vi "Convert Flow Data.vi"(8 "error in (no error)":errorcluster, 10 "register values - 3B":u16[](array[numeric]) format="%.0x", 11 "register values - 3A":u16[](array[numeric]) format="%.0x") -> (0 "error out":errorcluster, 3 "Flow Rate (SCFH)":dbl)   [LabVIEW 2020]
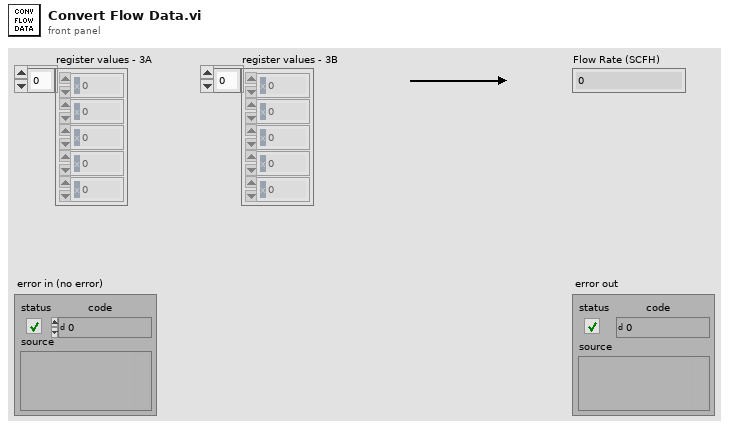
[diagram p1: front panel]
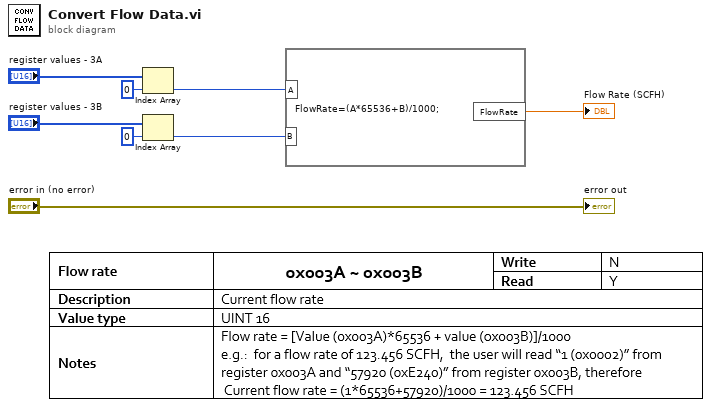
[diagram p0: block diagram]
diagram:
  n1 = Index Array(array="register values - 3A", index=0) -> (element=w3:u16)
  n2 = Index Array(array="register values - 3B", index=0) -> (element=w2:u16)
  n3 = formula code="FlowRate=(A*65536+B)/1000;"("A"=w3, "B"=w2) -> ("FlowRate"=→"Flow Rate (SCFH)":dbl)
  "error out" <- "error in (no error)"
